vi "2d_array_to_Javascript_2.vi"(5 "names":string[](array[string]), 7 "Array":dbl[][](array[numeric]), 10 "file path (use dialog)":path) -> (0 "web page write":errorcluster)   [LabVIEW 2013]
doc: "Saves the xy graph to a javascript file usable by mjs_plot.js."
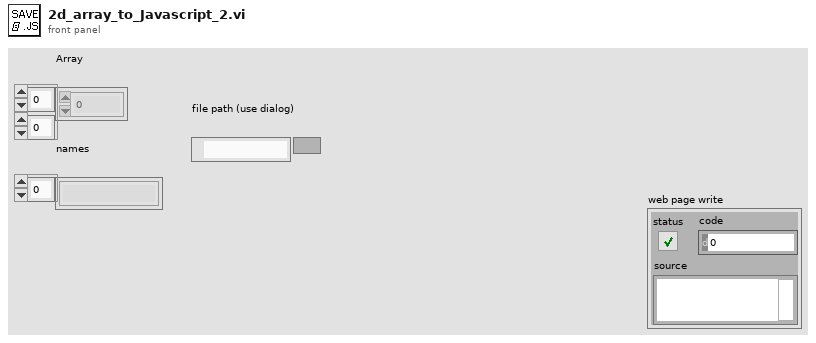
[diagram p1: front panel]
types:
  T1 = enum16{"open", "replace", "create", "open or create", "replace or create", "replace or create with confirmation"}
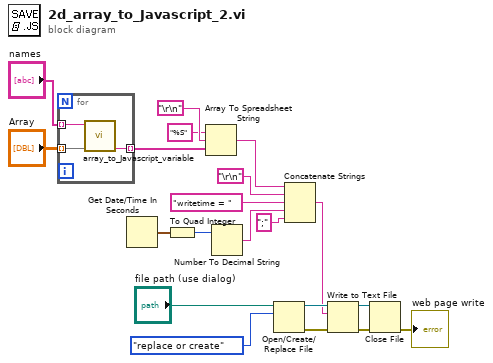
[diagram p0: block diagram]
diagram:
  n1 = for {
    tunnel: "Array" -> [w23] mode=indexing
    tunnel: "names" -> [w22] mode=indexing
    tunnel: [w21] -> w9 mode=indexing
    n2 = call "array_to_Javascript_variable.vi"("array"=w23, "variable_name"=w22) -> ("variable_string"=w21:string)  [unwired: 8 in]
  }
  n3 = Get Date/Time In Seconds() -> (seconds since 1Jan1904=w8:timestamp)
  n4 = To Quad Integer(1:w8) -> (0:w7:i64)
  n5 = Array To Spreadsheet String(delimiter (Tab)="\r\n", array=w9, 3:"%S" ("format string")) -> (spreadsheet string=w1:string)
  n6 = Number To Decimal String(number=w7) -> (decimal integer string=w5:string)  [unwired: 1 in]
  n7 = Open/Create/Replace File(file path (use dialog)="file path (use dialog)", operation (0:open)=T1."replace or create") -> (refnum out=w15:refnum<file>, error out=w12:errorcluster)  [unwired: 4 in, 1 out]
  n8 = Concatenate Strings(w1, "\r\n", "writetime = " ("string"), w5, ";" ("string")) -> (w3:string)
  n9 = Write to Text File(file (use dialog)=w15, text=w3, error in=w12) -> (refnum out=w14:refnum<file>, error out=w13:errorcluster)  [unwired: 1 in, 1 out]
  n10 = Close File(refnum=w14, error in=w13) -> (error out=→"web page write":errorcluster)  [unwired: 1 out]
